vi "Assert True.vi"(9 "Boolean ( True)":bool=TRUE) -> ()   [LabVIEW 2020, in "WebServiceImporter.lvlib" / "Error Handling.lvlib"]
uses:
  <vilib>/Platform/WebService/Error Handling/Error Handling.lvlib
  <vilib>/Platform/WebService/Error Handling/Assert/Assert Number.ctl
panel:
  in  "Assert Number":T1 items=["LabVIEW Internal Error"]
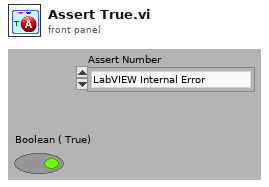
[diagram p1: front panel]
types:
  T1 = typedef "WebServiceImporter.lvlib/Error Handling.lvlib/Assert Number.ctl" = u16
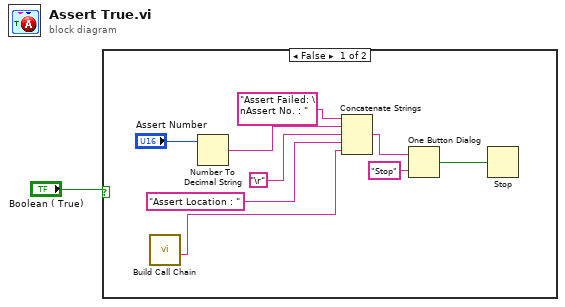
[diagram p0: block diagram]
diagram:
  n1 = case shown="False" "Boolean ( True)" {
    frame False {
      n2 = call <vilib>:"Build Call Chain.vi"() -> ("Call Chain"=w3:string)  [unwired: 11 in]
      n3 = Number To Decimal String(number="Assert Number") -> (decimal integer string=w6:string)  [unwired: 1 in]
      n4 = Concatenate Strings("Assert Failed: \nAssert No. : ", w6, "\r", "Assert Location : ", w3) -> (w2:string)
      n5 = One Button Dialog(message=w2, button name ("OK")="Stop") -> (true=w9:bool)
      n6 = Stop(stop? (T)=w9) -> ()
    }
    frame True {
    }
  }
